vi "Check data length_PortX.vi"(8 "error in":errorcluster, 11 "# samples in buffer":u16) -> (0 "error iout":errorcluster, 2 "Modbus Function":T1, 3 "# samples in buffer out":u16)   [LabVIEW 2022 SP3]
uses:
  Ctl/Modbus Function TCP.ctl
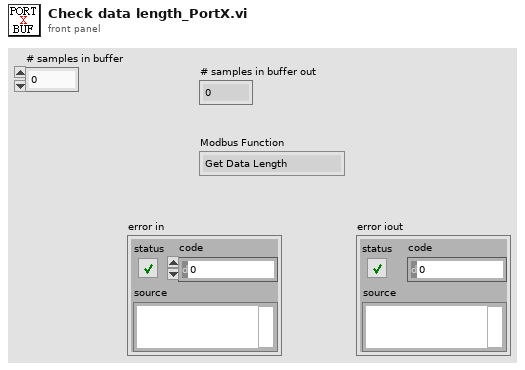
[diagram p1: front panel]
types:
  T1 = typedef "Modbus Function TCP.ctl" = enum16{"Get Data Length", "Normal Mode", "Bulk Mode", "Reconnect Port", "Recconect Box", "BoxReady"}
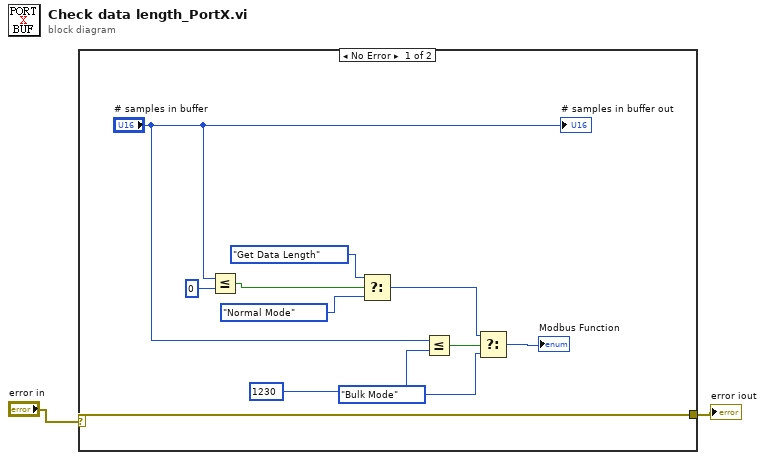
[diagram p0: block diagram]
diagram:
  n1 = case shown="No Error" "error in" {
    selector: "error in" -> [w3 w14]
    tunnel: [w3 w14] -> w1
    frame No Error {
      n2 = Less Or Equal?(x="# samples in buffer", y=u16 0) -> (x <= y?=w12:bool)
      n3 = Select(t=Modbus_Function_TCP."Get Data Length" ("Modbus"), s=w12, f=Modbus_Function_TCP."Normal Mode" ("Modbus")) -> (s? t:f=w8:T1)
      n4 = Less Or Equal?(x="# samples in buffer", y=u16 1230 ("bulk mode trigger (size)")) -> (x <= y?=w9:bool)
      n5 = Select(t=w8, s=w9, f=Modbus_Function_TCP."Bulk Mode" ("Modbus")) -> (s? t:f=→"Modbus Function":T1)
      "# samples in buffer out" <- "# samples in buffer"
    }
    frame Error {
    }
  }
  "error iout" <- w1
